vi "GetType.vi"(8 "error in (no error)":errorcluster, 11 "Set Ratio Msg":refnum<class "Set Ratio Msg.lvclass">) -> (0 "error out":errorcluster, 2 "Data Sample":variant, 3 "Set Ratio Msg":refnum<class "Set Ratio Msg.lvclass">)   [LabVIEW 2021, in "BNT_ULx.lvlib" / "Set Ratio Msg.lvclass"]
uses:
  Set Ratio Msg.lvclass
  Set Ratio Msg.lvclass/Set Ratio Msg.ctl
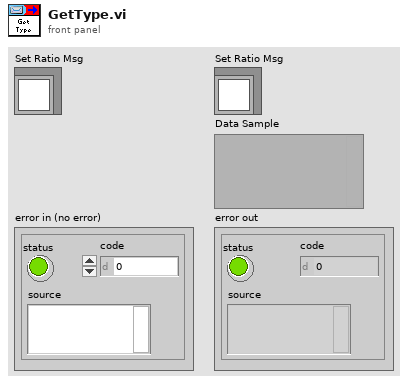
[diagram p1: front panel]
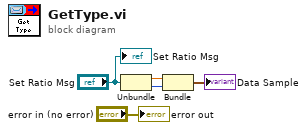
[diagram p0: block diagram]
diagram:
  n1 = Unbundle("Set Ratio Msg") -> (w2:dbl, w1:i32)
  n2 = Bundle("PWM Ratio"=w2, "Line"=w1) -> (→"Data Sample":cluster{"PWM Ratio":dbl, "Line":i32})  [unwired: 1 in]
  "error out" <- "error in (no error)"
  "Set Ratio Msg" <- "Set Ratio Msg"
